vi "dBResta.vi"(3 "Potencia Salida":dbl, 4 "error in (no error)":errorcluster, 5 "Potencia Entrada":dbl) -> (0 "error out":errorcluster, 1 "dB":dbl)   [LabVIEW 2019]
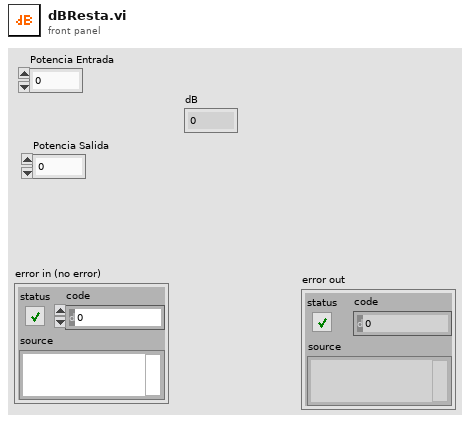
[diagram p1: front panel]
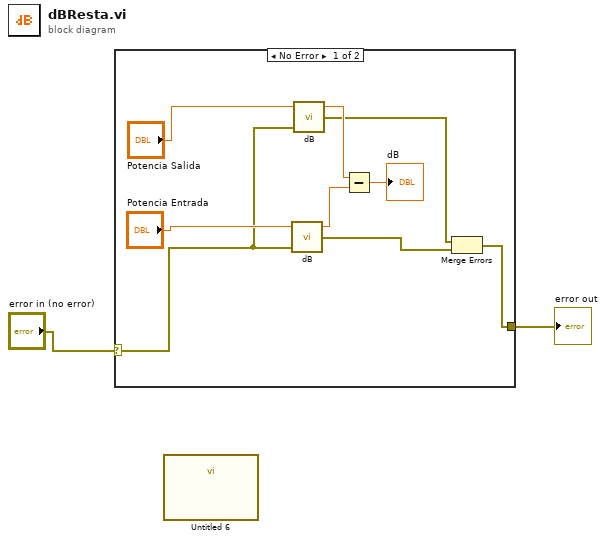
[diagram p0: block diagram]
diagram:
  n1 = case shown="No Error" "error in (no error)" {
    selector: "error in (no error)" -> [w8 w12]
    tunnel: [w3 w12] -> w1
    frame No Error {
      n2 = call "dB.vi"("error in (no error)"=w8, "Potencia"="Potencia Entrada") -> ("error out"=w4:errorcluster, "dBW"=w6:dbl)  [unwired: 1 in, 1 out]
      n3 = call "dB.vi"("error in (no error)"=w8, "Potencia"="Potencia Salida") -> ("error out"=w5:errorcluster, "dBW"=w7:dbl)  [unwired: 1 in, 1 out]
      n4 = Subtract(x=w7, y=w6) -> (x-y=→"dB":dbl)
      n5 = Merge Errors(w5, w4) -> (w3:errorcluster)
    }
    frame Error {
    }
  }
  "error out" <- w1
  n6 = call "Untitled 6.vi"() -> ()  [unwired: 14 in, 2 out]
